vi "xc calculator.vi"(9 "Z":dbl, 10 "Y":dbl, 11 "X":dbl) -> (2 "xc":dbl)   [LabVIEW 2014, in "AMS TS3472 Light Sensor.lvlib" / "AMS TCS3472.lvclass"]
uses:
  AMS TCS3472.lvclass
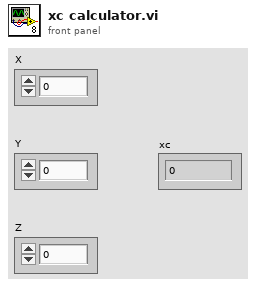
[diagram p1: front panel]
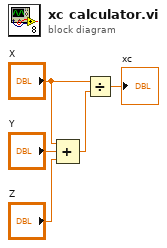
[diagram p0: block diagram]
diagram:
  n1 = Compound Arithmetic op=ADD("X", "Y", "Z") -> (w5:dbl)
  n2 = Divide(x="X", y=w5) -> (x/y=→"xc":dbl)
